vi "UpdateConfiguration.vi"(2 "error in (no error)":errorcluster, 3 "INSTR_PARAM.Config":T1={"IntTime"=100, "Samples"=3, "PowerMin"=400.0, "KneeMin"=-20.0, "KneeMax"=20.0, "Background Wl"=275.0, "Settle Delay,ms"=275, "StationId"=0.0} {"Background Wl" min=220.0 max=320.0; "IntTime" min=1 max=100000; "Samples" min=1 max=10; "PowerMin" min=0.0 max=10000.0; "KneeMin" min=-40.0 max=0.0; "KneeMax" min=0.0 max=40.0}, 4 "Instruments in":refnum<class "Instruments.lvclass">) -> (0 "error out":errorcluster, 1 "Instruments out":refnum<class "Instruments.lvclass">)   [LabVIEW 2012, in "Instruments.lvclass"]
uses:
  Instruments.lvclass
  Controls/Config.ctl
  Instruments.lvclass/Instruments.ctl
panel:
  # "Measurement Settings"
  # "Test Criteria"
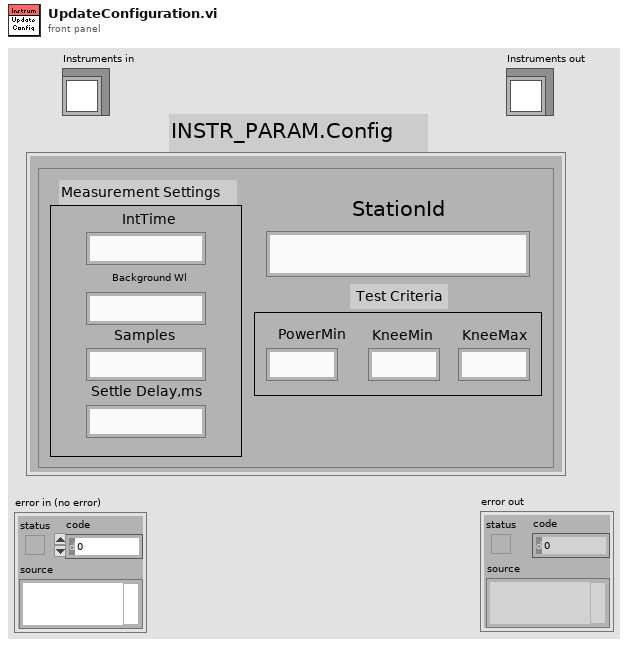
[diagram p1: front panel]
types:
  T1 = typedef "Config.ctl" = cluster{"IntTime":i32, "Samples":i32, "PowerMin":dbl, "KneeMin":dbl, "KneeMax":dbl, "Background Wl":dbl, "Settle Delay,ms":u32, "StationId":sgl}
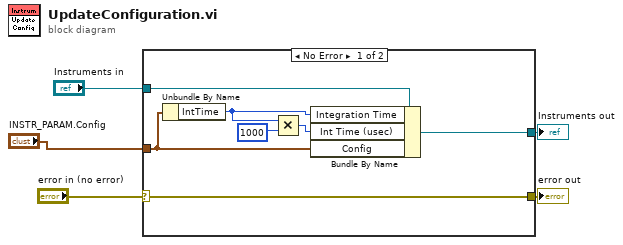
[diagram p0: block diagram]
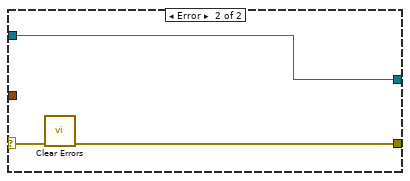
[diagram p2: hidden frame]
diagram:
  n1 = case shown="No Error" "error in (no error)" {
    selector: "error in (no error)" -> [w7 w14]
    tunnel: [w7 w13] -> w4
    tunnel: [w8 w15] -> w2
    tunnel: "Instruments in" -> [w12 w15]
    tunnel: "INSTR_PARAM.Config" -> [w6 _]
    frame No Error {
      n2 = Unbundle By Name(w6) -> ("IntTime"=w10:i32)
      n3 = Multiply(x=w10, y=1000) -> (x*y=w9:i32)
      n4 = Bundle By Name(cluster=w12, "Integration Time"=w10, "Int Time (usec)"=w9, "Config"=w6) -> (w8:refnum<class "Instruments.lvclass">)
    }
    frame Error {
      n5 = call <vilib>:"Clear Errors.vi"("error in (no error)"=w14) -> ("error out"=w13:errorcluster)  [unwired: 6 in]
    }
  }
  "error out" <- w4
  "Instruments out" <- w2
